vi "VerifyArguments.vi"(8 "error in (no error)":errorcluster, 11 "DiffVI in":refnum<class "DiffVI.lvclass">) -> (0 "error out":errorcluster, 3 "DiffVI out":refnum<class "DiffVI.lvclass">)   [LabVIEW 2015, in "DiffVI.lvclass"]
uses:
  DiffVI.lvclass
  DiffVI.lvclass/DiffVI.ctl
  <nishared>/LabVIEW CLI/Operations/Utilities/OperationErrorType.ctl
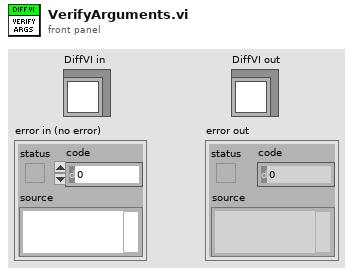
[diagram p1: front panel]
types:
  T1 = typedef "OperationErrorType.ctl" = enum16{"RequiredArgumentMissing", "UnknownArguments", "LoggerSetMultipleTimes", "OperationBrokenError"}
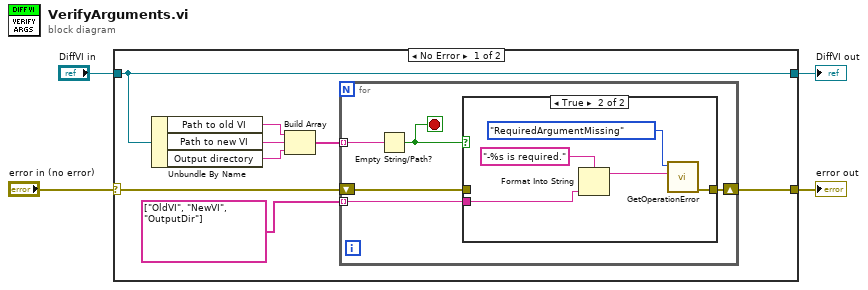
[diagram p0: block diagram]
diagram:
  n1 = case shown="No Error" "error in (no error)" {
    selector: "error in (no error)" -> [w12 w25]
    tunnel: [w11 w25] -> w2
    tunnel: [w10 w24] -> w3
    tunnel: "DiffVI in" -> [w10 w24]
    frame No Error {
      n2 = Unbundle By Name(w10) -> ("Path to old VI"=w8:string, "Path to new VI"=w7:string, "Output directory"=w6:string)
      n3 = Build Array(w8, w7, w6) -> (w5:string[])
      n4 = for {
        shift-right: [w16] -> w11
        shift-left: w12 -> [w17]
        tunnel: string[] ["OldVI", "NewVI", "OutputDir"] ("Additional Information") -> [w15] mode=indexing
        tunnel: w5 -> [w14] mode=indexing
        stop <- w13 stop-if-true
        n5 = Empty String/Path?(string/path=w14) -> (empty?=w13:bool)
        n6 = case shown="True" w13 {
          tunnel: w17 -> [w18 _]
          tunnel: [w18 w23] -> w16
          tunnel: w15 -> [_ w19]
          frame False {
          }
          frame True {
            n7 = Format Into String(format string="-%s is required.", w19) -> (resulting string=w20:string)  [unwired: 2 in, 1 out]
            n8 = call <nishared>:"GetOperationError.vi"("Additional Information"=w20, "Operation Error Type"=OperationErrorType."RequiredArgumentMissing") -> ("error out"=w23:errorcluster)  [unwired: 9 in]
          }
        }
      }
    }
    frame Error {
    }
  }
  "DiffVI out" <- w3
  "error out" <- w2
